vi "WaitAdjustTesting.vi"() -> ()   [LabVIEW 2019]
uses:
  <vilib>/numeric/Random Number (Range) I64.vi
  <vilib>/Rock Robotics/WPI/ThirdParty/JAS_Junk/TrajLib/LinearFilter_ResetToValue.vi
  <vilib>/Rock Robotics/WPI/ThirdParty/JAS_Junk/TrajLib/LinearFilter_Calculate.vi
  <vilib>/Rock Robotics/WPI/ThirdParty/JAS_Junk/TrajLib/MathUtil_Clamp.vi
  <vilib>/numeric/sub_Random U32.vi
  <vilib>/Rock Robotics/WPI/ThirdParty/JAS_Junk/TrajLib/LinearFilter_MovingAverage.vi
  <vilib>/Rock Robotics/WPI/ThirdParty/JAS_Junk/TrajLib/LinearFilter_LowPassBW1.vi
  <vilib>/Rock Robotics/WPI/ThirdParty/JAS_Junk/TrajLib/LinearFilter_LowPassBW2.vi
  <vilib>/Rock Robotics/WPI/ThirdParty/JAS_Junk/TrajLib/LinearFilter_HighPassBW1.vi
  <vilib>/Rock Robotics/WPI/ThirdParty/JAS_Junk/TrajLib/LinearFilter_HighPassBW2.vi
  <vilib>/Rock Robotics/WPI/ThirdParty/JAS_Junk/TrajLib/Trajectory_Library.lvlib
  <vilib>/gmath/NI_AAL_MathFunc.lvlib
panel:
  out "Deviation 2":dbl format="%13.5f"
  out "Deviation":dbl format="%13.5f"
  out "Time Diff":dbl
  out "AdjustedWaitTime_MS":u32
  out "Offset_MS":dbl
  out "Waveform Chart 2":dbl(graph)
  out "Waveform Chart":dbl(graph)
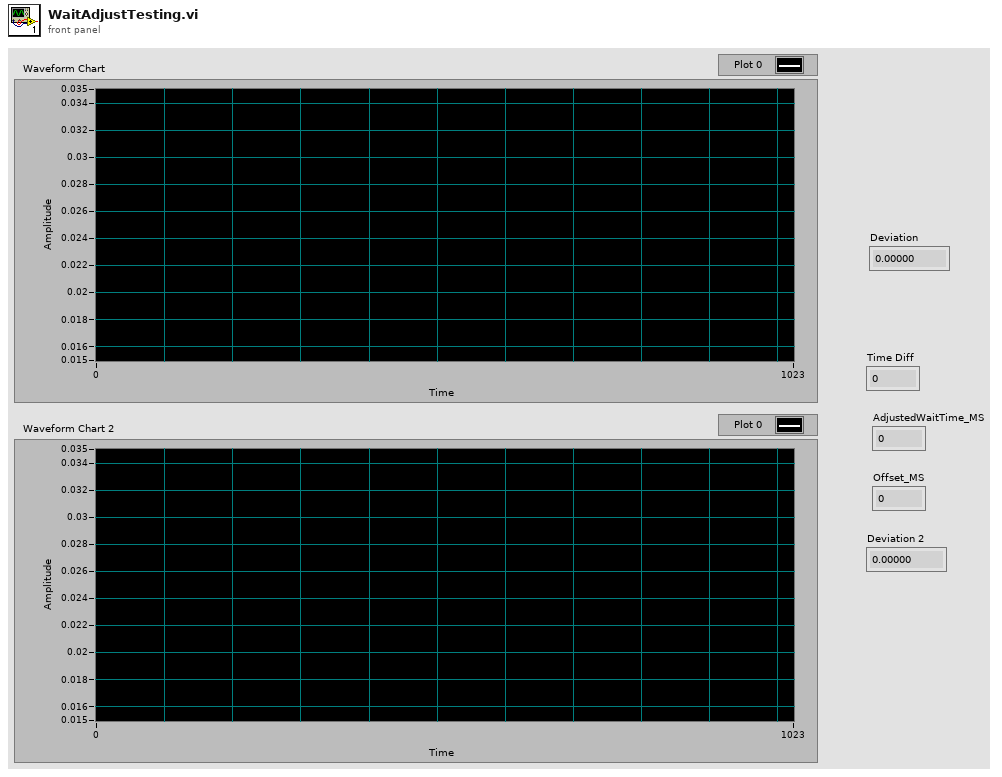
[diagram p1: front panel]
types:
  T1 = enum16{"Moving Average", "Low Pass 1st Order Butterworth", "Low Pass 2nd Order Butterworth", "High Pass 1st Order Butterworth", "High Pass 2nd Order Butterworth"}
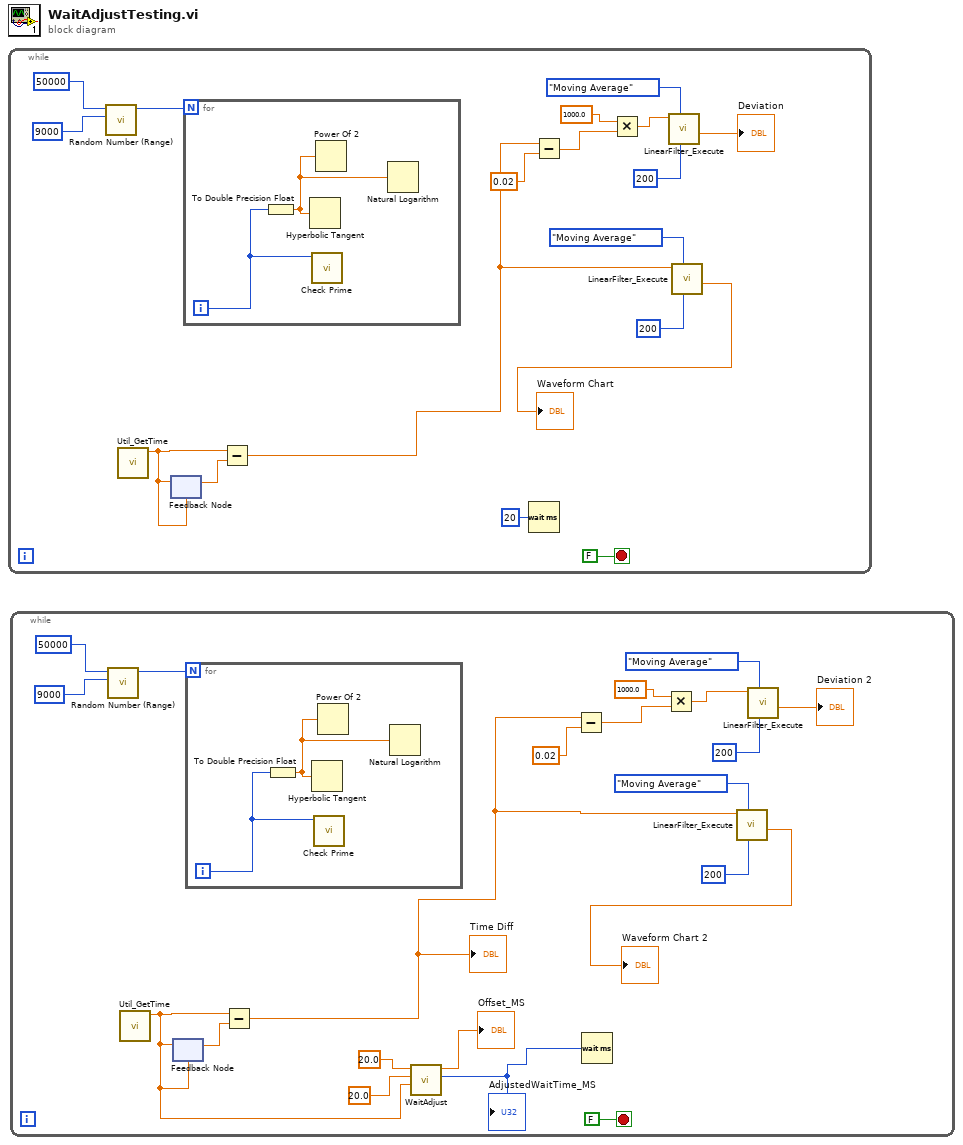
[diagram p0: block diagram]
diagram:
  n1 = while {
    stop <- FALSE stop-if-true
    n2 = call-poly <vilib>:"Random Number (Range).vi"("lower bound (-100)"=u64 9000 ("lower bound (0)"), "upper bound (100)"=u64 50000) -> ("number"=w13:i64)  [unwired: 9 in]
    n3 = call <vilib>:"Util_GetTime.vi"() -> ("FPGA_Time_Seconds"=w12:dbl)  [unwired: 10 in, 1 out]
    n4 = feedback-in #1(w12) -> ()
    n5 = feedback #1(w12) -> (w18:dbl)
    n6 = for {
      N: w13 -> [_]
      i -> [w20]
      n7 = To Double Precision Float(number=w20) -> (double precision float=w19:dbl)
      n8 = Hyperbolic Tangent(1:w19) -> ()  [unwired: 1 out]
      n9 = call <vilib>:"Check Prime.vi"("n"=w20) -> ()  [unwired: 10 in, 1 out]
      n10 = Power Of 2(x=w19) -> ()  [unwired: 1 out]
      n11 = Natural Logarithm(1:w19) -> ()  [unwired: 1 out]
    }
    n12 = Subtract(x=w12, y=w18) -> (x-y=w6:dbl)
    n13 = Wait (ms)(milliseconds to wait=u32 20) -> ()  [unwired: 1 out]
    n14 = Subtract(x=w6, y=0.02) -> (x-y=w2:dbl)
    n15 = Multiply(x=1000.0, y=w2) -> (x*y=w3:dbl)
    n16 = call <vilib>:"LinearFilter_Execute.vi"("Samples"=200, "Filter Type"=T1."Moving Average", "Input"=w3) -> ("Output"=→"Deviation":dbl)  [unwired: 7 in, 1 out]
    n17 = call <vilib>:"LinearFilter_Execute.vi"("Samples"=200, "Filter Type"=T1."Moving Average", "Input"=w6) -> ("Output"=→"Waveform Chart":dbl)  [unwired: 7 in, 1 out]
  }
  n18 = while {
    stop <- FALSE stop-if-true
    n19 = call-poly <vilib>:"Random Number (Range).vi"("lower bound (-100)"=u64 9000 ("lower bound (0)"), "upper bound (100)"=u64 50000) -> ("number"=w37:i64)  [unwired: 9 in]
    n20 = call <vilib>:"Util_GetTime.vi"() -> ("FPGA_Time_Seconds"=w33:dbl)  [unwired: 10 in, 1 out]
    n21 = feedback-in #2(w33) -> ()
    n22 = feedback #2(w33) -> (w41:dbl)
    n23 = for {
      N: w37 -> [_]
      i -> [w43]
      n24 = To Double Precision Float(number=w43) -> (double precision float=w42:dbl)
      n25 = Hyperbolic Tangent(1:w42) -> ()  [unwired: 1 out]
      n26 = call <vilib>:"Check Prime.vi"("n"=w43) -> ()  [unwired: 10 in, 1 out]
      n27 = Power Of 2(x=w42) -> ()  [unwired: 1 out]
      n28 = Natural Logarithm(1:w42) -> ()  [unwired: 1 out]
    }
    n29 = Subtract(x=w33, y=w41) -> (x-y=w24:dbl)
    "Time Diff" <- w24
    n30 = call <vilib>:"WaitAdjust.vi"("Time_SEC"=w33, "MaxDeviation_MS"=20.0, "DesiredLoopTime_MS"=20.0) -> ("AdjustedWaitTime_MS"=w36:u32, "Offset_MS"=→"Offset_MS":dbl)  [unwired: 7 in]
    "AdjustedWaitTime_MS" <- w36
    n31 = Subtract(x=w24, y=0.02) -> (x-y=w22:dbl)
    n32 = Wait (ms)(milliseconds to wait=w36) -> ()  [unwired: 1 out]
    n33 = Multiply(x=1000.0, y=w22) -> (x*y=w21:dbl)
    n34 = call <vilib>:"LinearFilter_Execute.vi"("Samples"=200, "Filter Type"=T1."Moving Average", "Input"=w24) -> ("Output"=→"Waveform Chart 2":dbl)  [unwired: 7 in, 1 out]
    n35 = call <vilib>:"LinearFilter_Execute.vi"("Samples"=200, "Filter Type"=T1."Moving Average", "Input"=w21) -> ("Output"=→"Deviation 2":dbl)  [unwired: 7 in, 1 out]
  }
